vi "Set_T.vi"(7 "Numeric":dbl) -> (3 "Numeric 2":dbl)   [LabVIEW 2016]
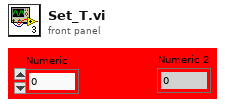
[diagram p1: front panel]
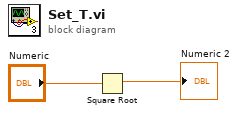
[diagram p0: block diagram]
diagram:
  n1 = Square Root(x="Numeric") -> (sqrt(x)=→"Numeric 2":dbl)
